vi "DeviceScan.vi"() -> ()   [LabVIEW 2017]
panel:
  out "VISA2":refnum<visa-resource-name>
  out "VISA1":refnum<visa-resource-name>
  out "substring 2":string
  out "substring":string
  out "text":string[](array[string])
  out "error out":errorcluster
  in  "error in (no error)":errorcluster
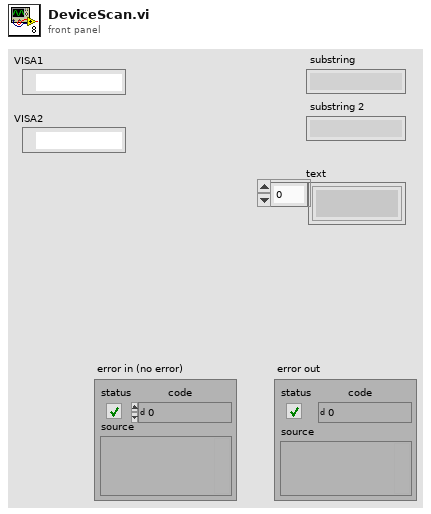
[diagram p1: front panel]
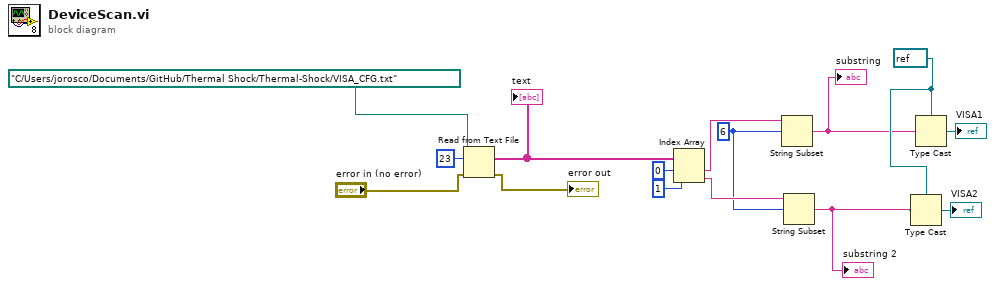
[diagram p0: block diagram]
diagram:
  w5 = refnum<visa-resource-name> refnum ("VISA resource name")
  w6 = 6 ("offset (0)")
  n1 = Read from Text File(file (use dialog)=path "C:/Users/jorosco/Documents/GitHub/Thermal Shock/Thermal-Shock/VISA_CFG.txt", count=23, error in="error in (no error)") -> (text=w11:string[], error out=→"error out":errorcluster)  [unwired: 1 in, 2 out]
  "text" <- w11
  n2 = Index Array(array=w11, index #1=0 ("index"), index #2=1 ("index")) -> (element #1=w8:string, element #2=w7:string)
  n3 = String Subset(string=w8, offset (0)=w6) -> (substring=w4:string)  [unwired: 1 in]
  "substring" <- w4
  n4 = String Subset(string=w7, offset (0)=w6) -> (substring=w3:string)  [unwired: 1 in]
  "substring 2" <- w3
  n5 = Type Cast(type=w5, x=w3) -> (*(type *) &x=→"VISA2":refnum<visa-resource-name>)
  n6 = Type Cast(type=w5, x=w4) -> (*(type *) &x=→"VISA1":refnum<visa-resource-name>)
